vi "Broadcast Position and Speed (Sub VI).vi"(8 "error in (no error)":errorcluster) -> (0 "error out":errorcluster)   [LabVIEW 2020, in "Manipulator.lvlib"]
uses:
  Manipulator.lvlib
  Get Position and Speed (Reply Payload)--cluster.ctl
  Manipulator-CLIDriver/Manipulator CLI Driver.lvlib
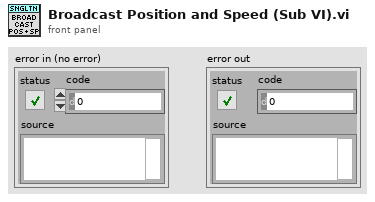
[diagram p1: front panel]
types:
  T1 = typedef "Manipulator.lvlib/Get Position and Speed (Reply Payload)--cluster.ctl" = cluster{"Positions":dbl[], "Speeds":dbl[], "Get Position and Speed_error":errorcluster}
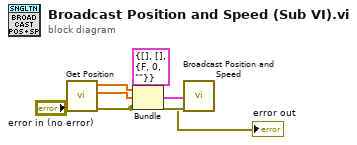
[diagram p0: block diagram]
diagram:
  n1 = call "Get Position.vi"("error in (no error)"="error in (no error)") -> ("error out"=w5:errorcluster, "speeds"=w6:dbl[], "positions"=w7:dbl[])  [unwired: 8 in]
  n2 = Bundle(cluster=T1 {"Positions"=[], "Speeds"=[], "Get Position and Speed_error"={"status"=FALSE, "code"=0, "source"=""}} ("Get Position and Speed (Reply Payload)"), "Positions"=w7, "Speeds"=w6, "Get Position and Speed_error"=w5) -> (w3:T1)
  n3 = call "Broadcast Position and Speed.vi"("error in"=w5, "Reply Payload"=w3) -> ("error out"=→"error out":errorcluster)  [unwired: 9 in]
